vi "Decode and Update.vi"(8 "error in":errorcluster, 9 "WiBCI16T Data":T1 {"Reg Map"."ADS2" format="%x"; "Reg Map"."ADS1" format="%x"}, 10 "data in":string, 11 "Data Valid ?":bool) -> (0 "error out":errorcluster, 3 "WiBCI16T Data out":T1 {"Reg Map"."ADS2" format="%x"; "Reg Map"."ADS1" format="%x"})   [LabVIEW 2019, in "Acquisition.lvlib"]
uses:
  Acquisition.lvlib
  WiBCI16T_Data.ctl
  WiBCI16T_Status.ctl
  Reg_Map.ctl
panel:
  out "substring":string
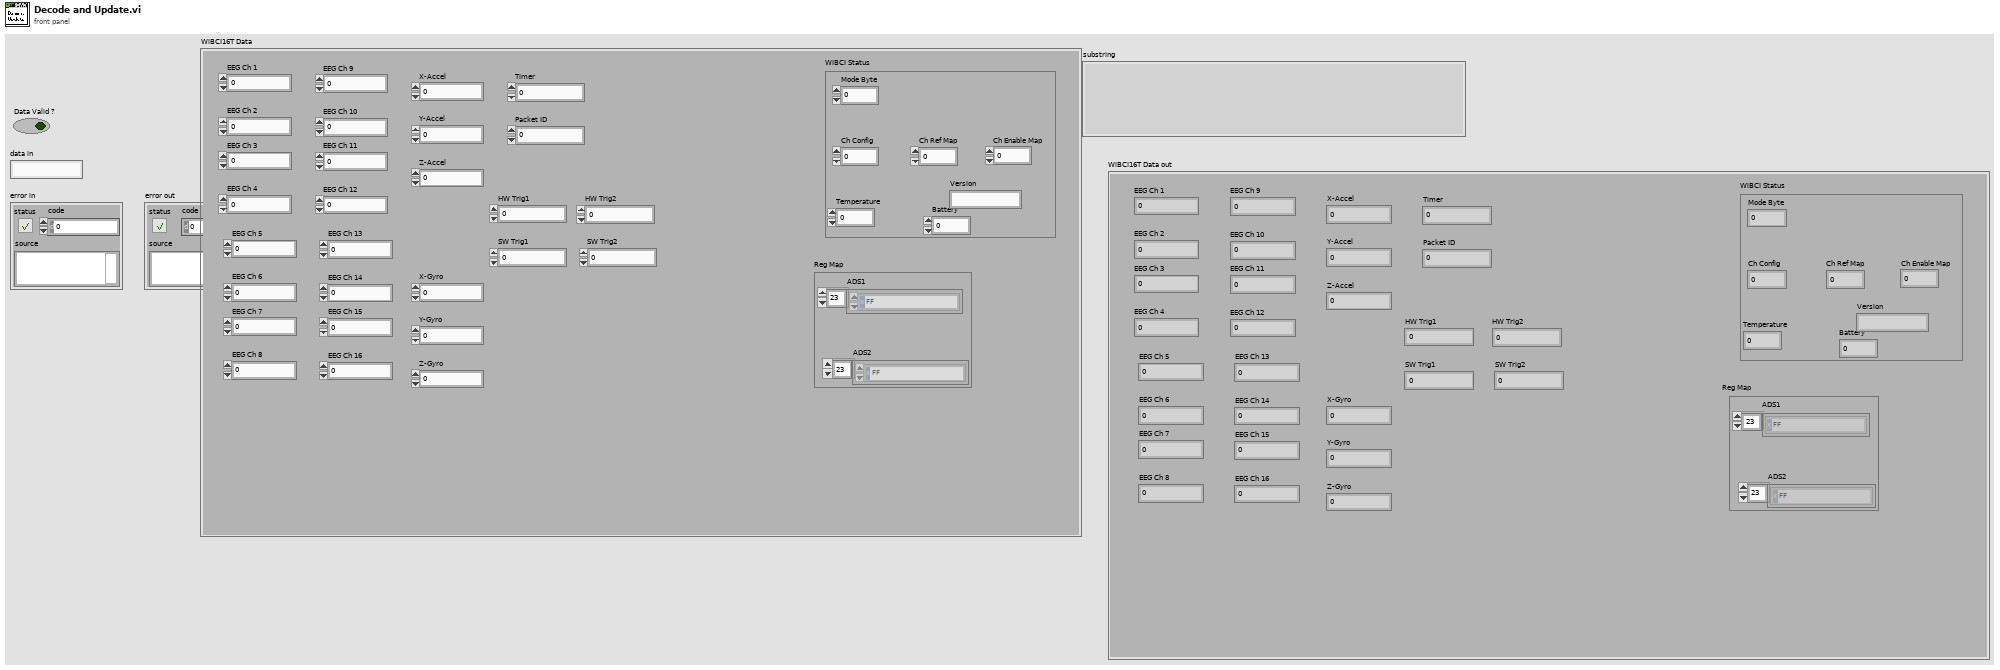
[diagram p1: front panel]
types:
  T1 = typedef "Acquisition.lvlib/WiBCI16T_Data.ctl" = cluster{"EEG Ch 1":dbl, "EEG Ch 2":dbl, "EEG Ch 3":dbl, "EEG Ch 4":dbl, "EEG Ch 5":dbl, "EEG Ch 6":dbl, "EEG Ch 7":dbl, "EEG Ch 8":dbl, "EEG Ch 9":dbl, "EEG Ch 10":dbl, "EEG Ch 11":dbl, "EEG Ch 12":dbl, "EEG Ch 13":dbl, "EEG Ch 14":dbl, "EEG Ch 15":dbl, "EEG Ch 16":dbl, "X-Accel":i16, "Y-Accel":i16, "Z-Accel":i16, "X-Gyro":i16, "Y-Gyro":i16, "Z-Gyro":i16, "Timer":u32, "Packet ID":u32, "HW Trig1":u8, "SW Trig1":i8, "HW Trig2":u8, "SW Trig2":i8, "WiBCI Status":T2, "Reg Map":T3}
  T2 = typedef "Acquisition.lvlib/WiBCI16T_Status.ctl" = cluster{"Mode Byte":u8, "Ch Config":u8, "Ch Ref Map":u16, "Ch Enable Map":u16, "Temperature":sgl, "Battery":u8, "Version":string}
  T3 = typedef "Acquisition.lvlib/Reg_Map.ctl" = cluster{"ADS1":u8[], "ADS2":u8[]}
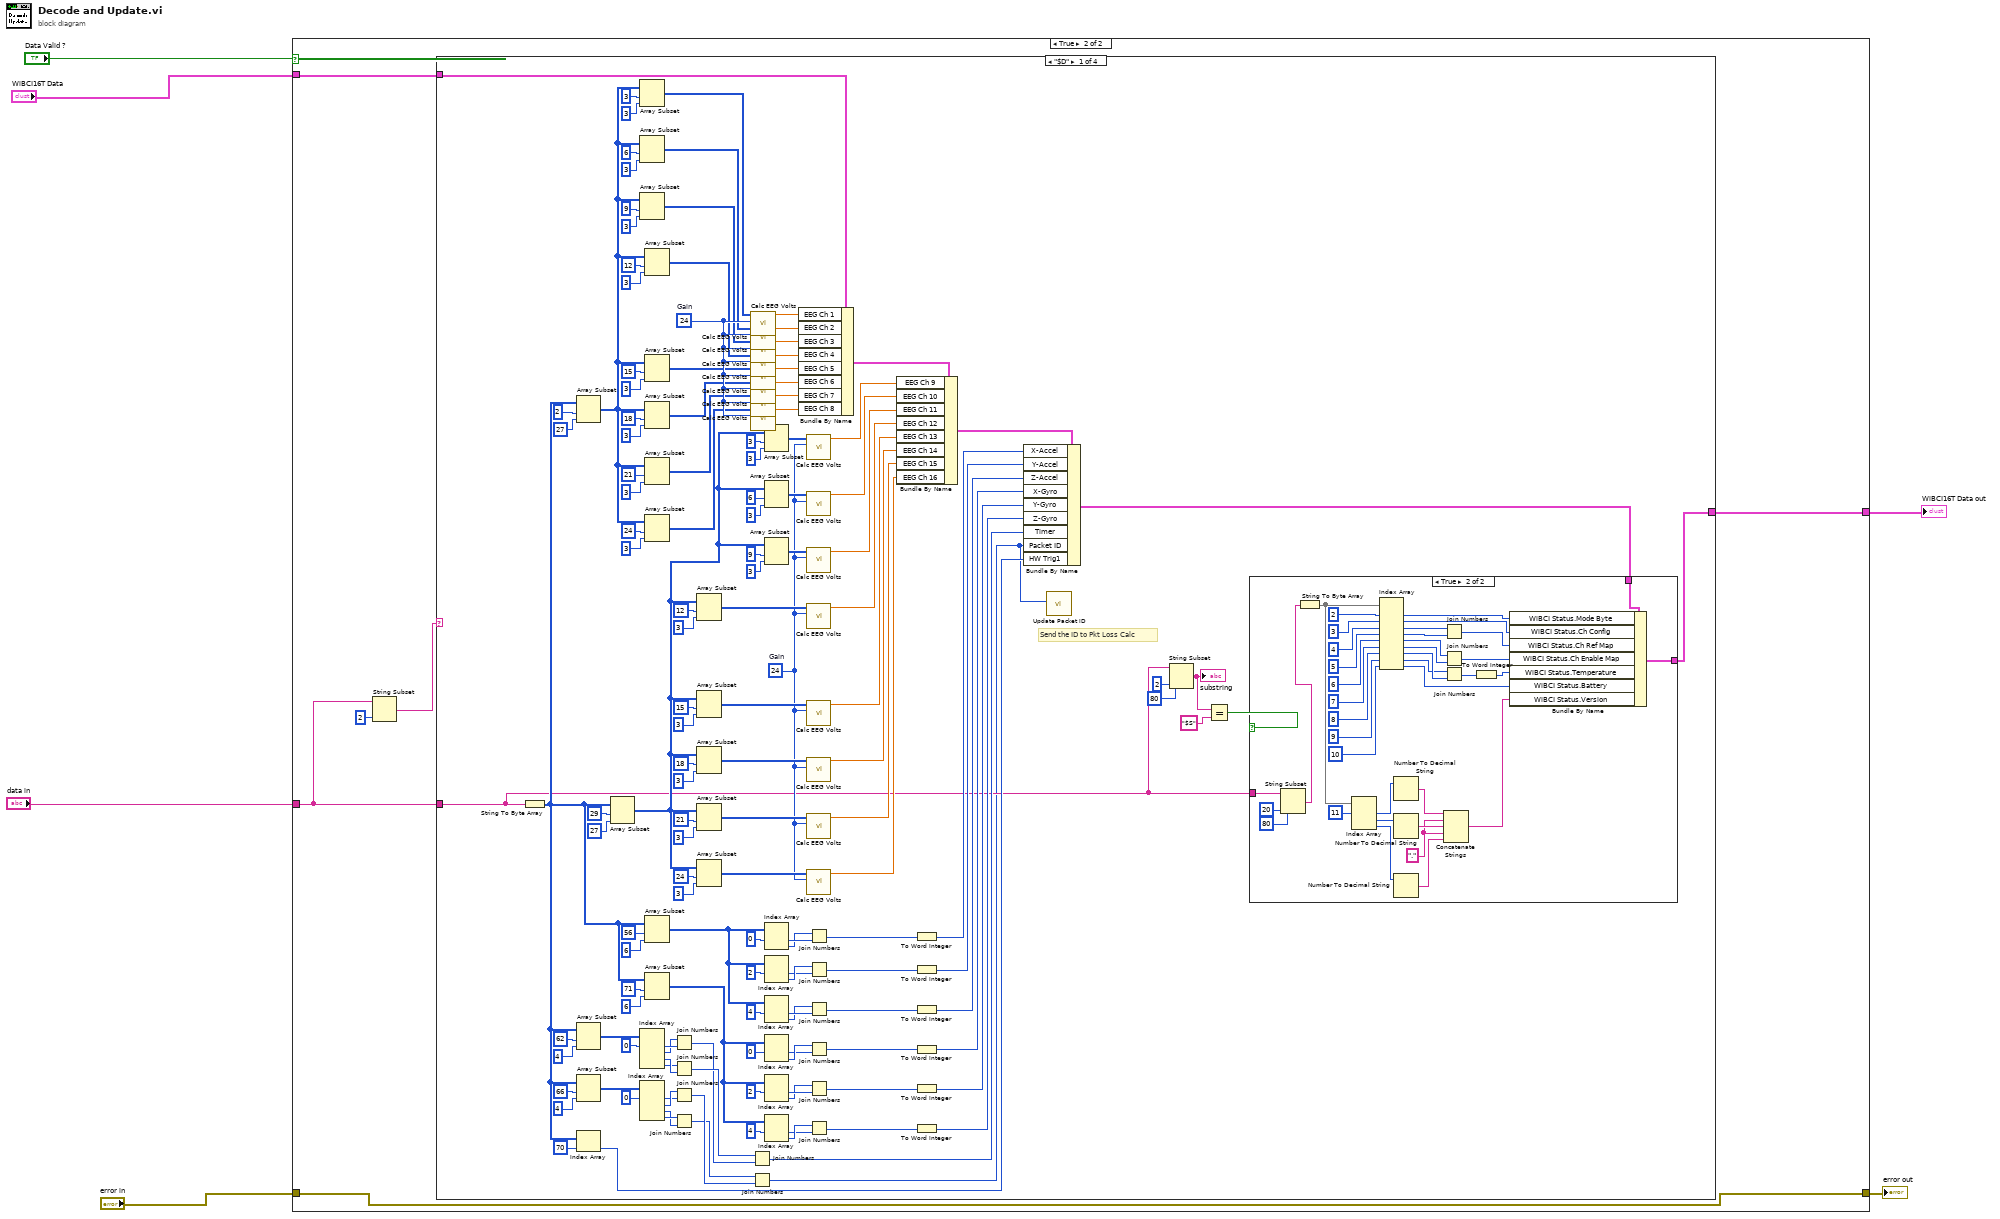
[diagram p0: block diagram]
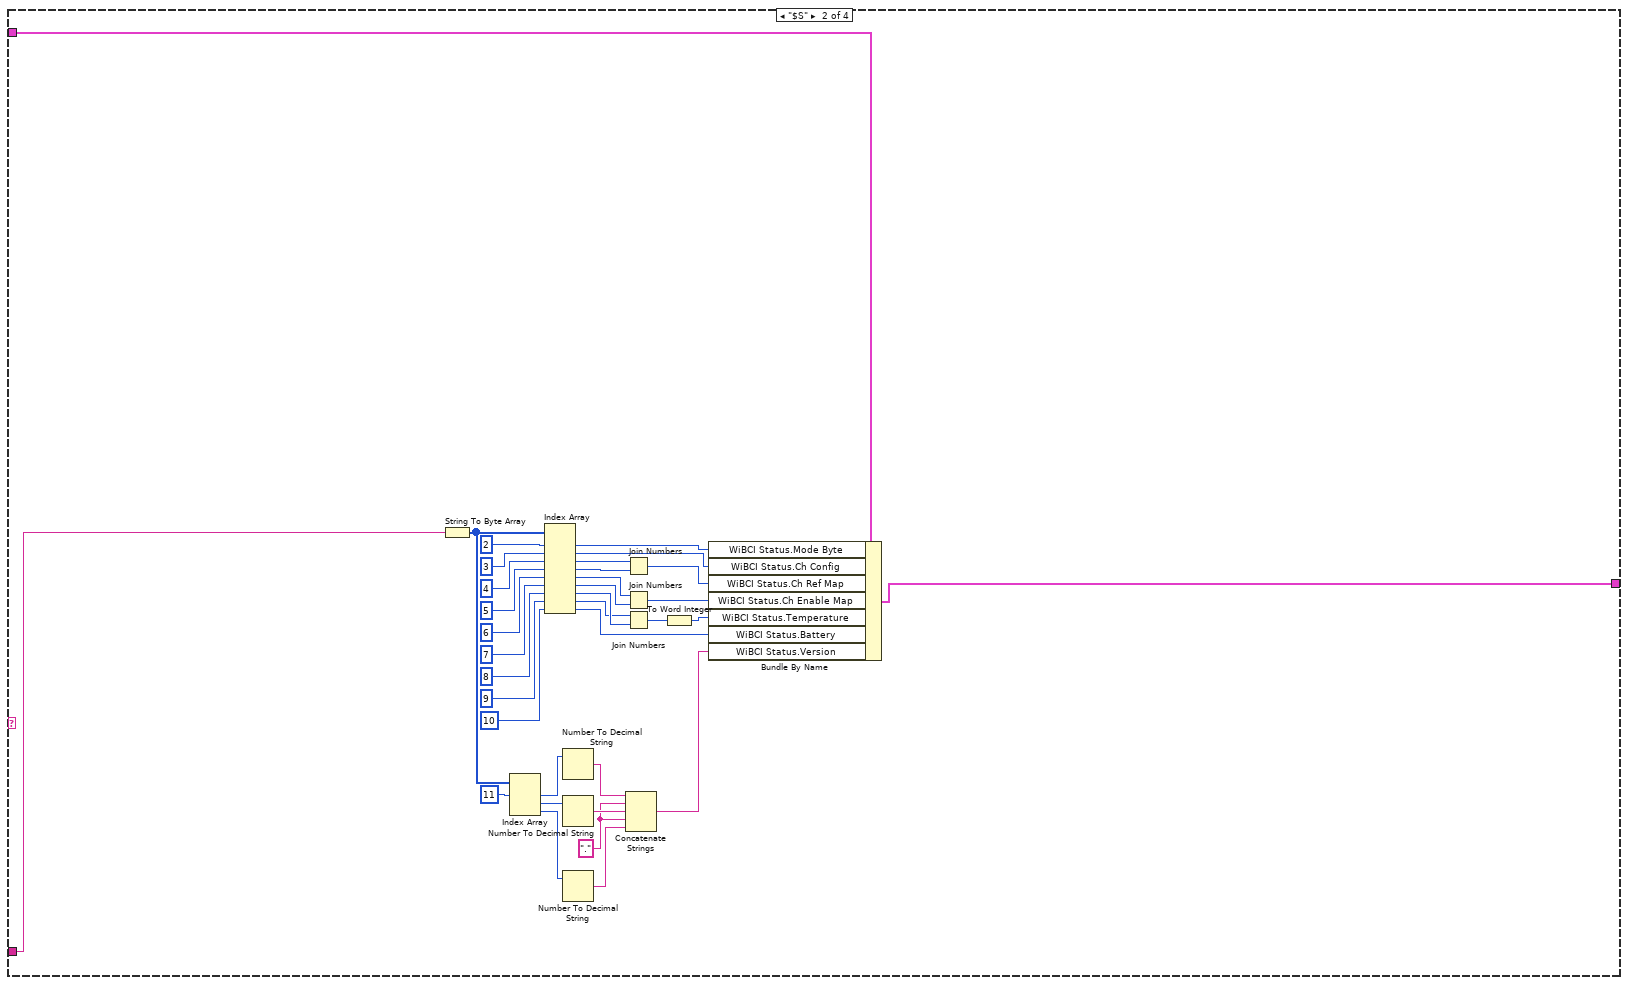
[diagram p4: hidden frame]
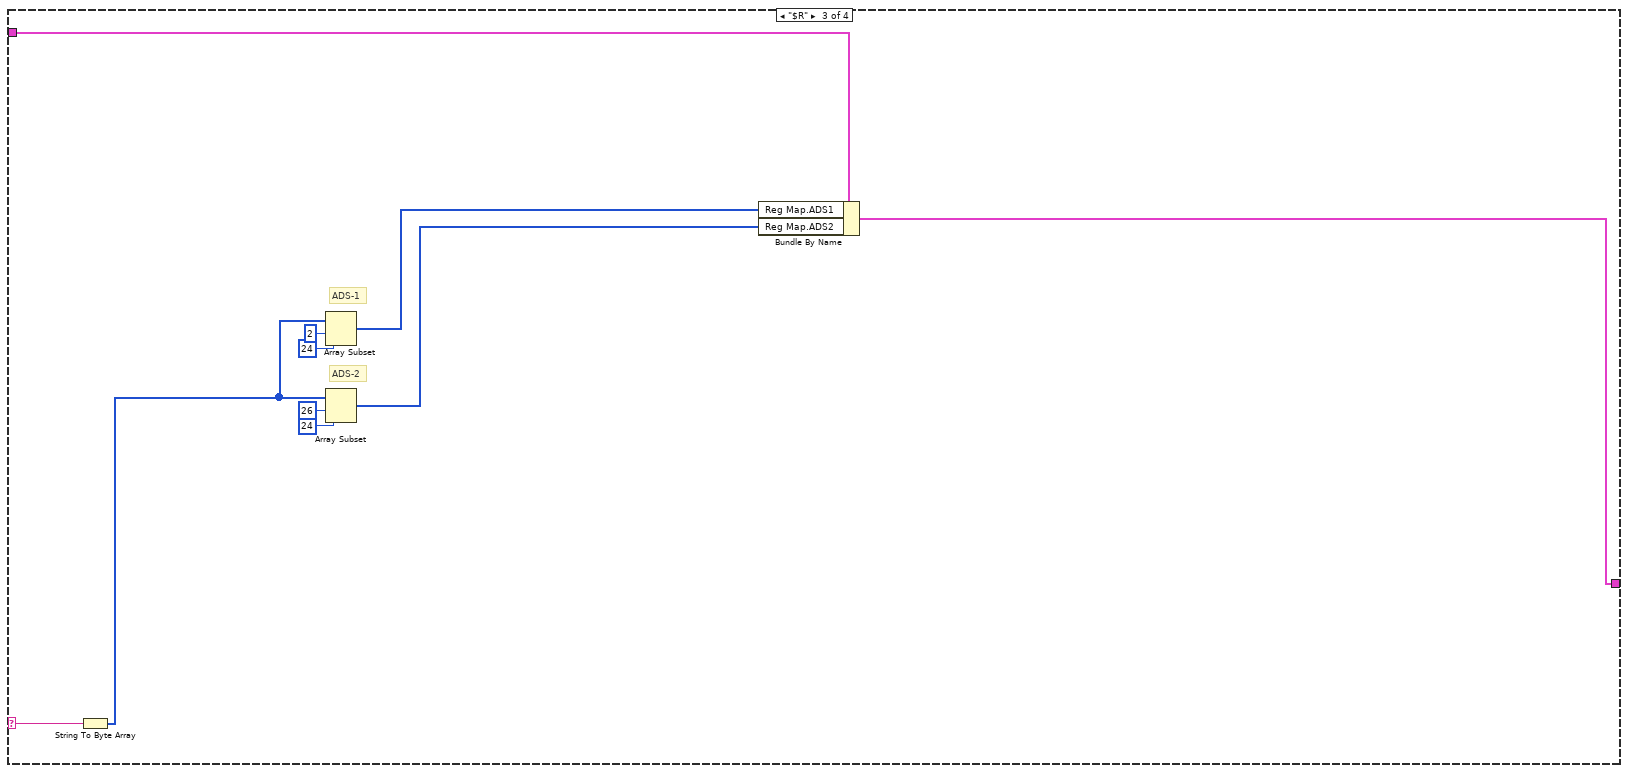
[diagram p5: hidden frame]
diagram:
  n1 = case shown="True" "Data Valid ?" {
    tunnel: "error in" -> [w8 w12]
    tunnel: [w8 w12] -> w5
    tunnel: "data in" -> [_ w10]
    tunnel: "WiBCI16T Data" -> [w7 w14]
    tunnel: [w7 w13] -> w1
    frame False {
    }
    frame True {
      n2 = String Subset(string=w10, length (rest)=2 ("length (rest)")) -> (substring=w9:string)  [unwired: 1 in]
      n3 = case shown="\"$D\"" w9 {
        selector: w9 -> [_ _ w236 _]
        tunnel: w14 -> [w128 w232 w242 w243]
        tunnel: [w16 w231 w241 w243] -> w13
        tunnel: w10 -> [w18 w198 _ _]
        frame "$D" {
          w103 = u8 24  # Gain
          w137 = u8 24  # Gain
          # "Send the ID to Pkt Loss Calc"
          n4 = String To Byte Array(string=w18) -> (unsigned byte array=w26:u8[])
          n5 = Array Subset(array=w26, index=2, length=27) -> (w138:u8[])
          n6 = Array Subset(array=w26, index=62, length=4) -> (w45:u8[])
          n7 = Array Subset(array=w26, index=66, length=4) -> (w30:u8[])
          n8 = Index Array(array=w26, index=70) -> (element=w24:u8)
          n9 = Array Subset(array=w26, index=29, length=27) -> (w85:u8[])
          n10 = Array Subset(array=w138, index=3, length=3) -> (w136:u8[])
          n11 = Array Subset(array=w138, index=6, length=3) -> (w135:u8[])
          n12 = Array Subset(array=w138, index=9, length=3) -> (w134:u8[])
          n13 = Index Array(array=w45, index #1=0 ("index")) -> (element #1=w43:u8, element #2=w42:u8, element #3=w41:u8, element #4=w40:u8)  [unwired: 3 in]
          n14 = Index Array(array=w30, index #1=0 ("index")) -> (element #1=w32:u8, element #2=w33:u8, element #3=w34:u8, element #4=w35:u8)  [unwired: 3 in]
          n15 = Array Subset(array=w138, index=12, length=3) -> (w133:u8[])
          n16 = Array Subset(array=w138, index=15, length=3) -> (w132:u8[])
          n17 = Array Subset(array=w138, index=18, length=3) -> (w131:u8[])
          n18 = Array Subset(array=w138, index=21, length=3) -> (w130:u8[])
          n19 = Array Subset(array=w138, index=24, length=3) -> (w129:u8[])
          n20 = Array Subset(array=w26, index=56, length=6) -> (w69:u8[])
          n21 = Array Subset(array=w26, index=71, length=6) -> (w65:u8[])
          n22 = Join Numbers(hi=w42, lo=w43) -> ((hi.lo)=w38:u16)
          n23 = Join Numbers(hi=w40, lo=w41) -> ((hi.lo)=w39:u16)
          n24 = Join Numbers(hi=w33, lo=w32) -> ((hi.lo)=w37:u16)
          n25 = Join Numbers(hi=w35, lo=w34) -> ((hi.lo)=w36:u16)
          n26 = Array Subset(array=w85, index=12, length=3) -> (w107:u8[])
          n27 = Array Subset(array=w85, index=15, length=3) -> (w108:u8[])
          n28 = Array Subset(array=w85, index=18, length=3) -> (w109:u8[])
          n29 = Array Subset(array=w85, index=21, length=3) -> (w110:u8[])
          n30 = Array Subset(array=w85, index=24, length=3) -> (w111:u8[])
          n31 = Join Numbers(hi=w39, lo=w38) -> ((hi.lo)=w27:u32)
          n32 = Join Numbers(hi=w36, lo=w37) -> ((hi.lo)=w15:u32)
          n33 = call "Calc EEG Volts.vi"("Gain"=w137, "Array"=w136) -> ("Volts"=w127:dbl)  [unwired: 9 in]
          n34 = call "Calc EEG Volts.vi"("Gain"=w137, "Array"=w135) -> ("Volts"=w126:dbl)  [unwired: 9 in]
          n35 = call "Calc EEG Volts.vi"("Gain"=w137, "Array"=w134) -> ("Volts"=w125:dbl)  [unwired: 9 in]
          n36 = call "Calc EEG Volts.vi"("Gain"=w137, "Array"=w133) -> ("Volts"=w124:dbl)  [unwired: 9 in]
          n37 = call "Calc EEG Volts.vi"("Gain"=w137, "Array"=w132) -> ("Volts"=w123:dbl)  [unwired: 9 in]
          n38 = call "Calc EEG Volts.vi"("Gain"=w137, "Array"=w131) -> ("Volts"=w122:dbl)  [unwired: 9 in]
          n39 = call "Calc EEG Volts.vi"("Gain"=w137, "Array"=w130) -> ("Volts"=w121:dbl)  [unwired: 9 in]
          n40 = call "Calc EEG Volts.vi"("Gain"=w137, "Array"=w129) -> ("Volts"=w120:dbl)  [unwired: 9 in]
          n41 = Array Subset(array=w85, index=3, length=3) -> (w104:u8[])
          n42 = Array Subset(array=w85, index=6, length=3) -> (w105:u8[])
          n43 = Array Subset(array=w85, index=9, length=3) -> (w106:u8[])
          n44 = Index Array(array=w69, index #1=0 ("index")) -> (element #1=w80:u8, element #2=w79:u8)  [unwired: 1 in]
          n45 = Index Array(array=w69, index #1=2 ("index")) -> (element #1=w75:u8, element #2=w76:u8)  [unwired: 1 in]
          n46 = Index Array(array=w69, index #1=4 ("index")) -> (element #1=w72:u8, element #2=w71:u8)  [unwired: 1 in]
          n47 = Index Array(array=w65, index #1=0 ("index")) -> (element #1=w54:u8, element #2=w55:u8)  [unwired: 1 in]
          n48 = Index Array(array=w65, index #1=2 ("index")) -> (element #1=w59:u8, element #2=w58:u8)  [unwired: 1 in]
          n49 = Index Array(array=w65, index #1=4 ("index")) -> (element #1=w62:u8, element #2=w63:u8)  [unwired: 1 in]
          n50 = Bundle By Name(cluster=w128, "EEG Ch 1"=w127, "EEG Ch 2"=w126, "EEG Ch 3"=w125, "EEG Ch 4"=w124, "EEG Ch 5"=w123, "EEG Ch 6"=w122, "EEG Ch 7"=w121, "EEG Ch 8"=w120) -> (w86:T1)
          n51 = call "Calc EEG Volts.vi"("Gain"=w103, "Array"=w104) -> ("Volts"=w112:dbl)  [unwired: 9 in]
          n52 = call "Calc EEG Volts.vi"("Gain"=w103, "Array"=w105) -> ("Volts"=w113:dbl)  [unwired: 9 in]
          n53 = call "Calc EEG Volts.vi"("Gain"=w103, "Array"=w106) -> ("Volts"=w114:dbl)  [unwired: 9 in]
          n54 = call "Calc EEG Volts.vi"("Gain"=w103, "Array"=w107) -> ("Volts"=w115:dbl)  [unwired: 9 in]
          n55 = call "Calc EEG Volts.vi"("Gain"=w103, "Array"=w108) -> ("Volts"=w116:dbl)  [unwired: 9 in]
          n56 = call "Calc EEG Volts.vi"("Gain"=w103, "Array"=w109) -> ("Volts"=w117:dbl)  [unwired: 9 in]
          n57 = call "Calc EEG Volts.vi"("Gain"=w103, "Array"=w110) -> ("Volts"=w118:dbl)  [unwired: 9 in]
          n58 = call "Calc EEG Volts.vi"("Gain"=w103, "Array"=w111) -> ("Volts"=w119:dbl)  [unwired: 9 in]
          n59 = Join Numbers(hi=w79, lo=w80) -> ((hi.lo)=w78:u16)
          n60 = Join Numbers(hi=w76, lo=w75) -> ((hi.lo)=w77:u16)
          n61 = Join Numbers(hi=w71, lo=w72) -> ((hi.lo)=w70:u16)
          n62 = Join Numbers(hi=w55, lo=w54) -> ((hi.lo)=w56:u16)
          n63 = Join Numbers(hi=w58, lo=w59) -> ((hi.lo)=w57:u16)
          n64 = Join Numbers(hi=w63, lo=w62) -> ((hi.lo)=w64:u16)
          n65 = Bundle By Name(cluster=w86, "EEG Ch 9"=w112, "EEG Ch 10"=w113, "EEG Ch 11"=w114, "EEG Ch 12"=w115, "EEG Ch 13"=w116, "EEG Ch 14"=w117, "EEG Ch 15"=w118, "EEG Ch 16"=w119) -> (w84:T1)
          n66 = To Word Integer(number=w78) -> (16bit integer=w68:i16)
          n67 = To Word Integer(number=w77) -> (16bit integer=w67:i16)
          n68 = To Word Integer(number=w70) -> (16bit integer=w66:i16)
          n69 = To Word Integer(number=w56) -> (16bit integer=w50:i16)
          n70 = To Word Integer(number=w57) -> (16bit integer=w49:i16)
          n71 = To Word Integer(number=w64) -> (16bit integer=w48:i16)
          n72 = Bundle By Name(cluster=w84, "X-Accel"=w68, "Y-Accel"=w67, "Z-Accel"=w66, "X-Gyro"=w50, "Y-Gyro"=w49, "Z-Gyro"=w48, "Timer"=w27, "Packet ID"=w15, "HW Trig1"=w24) -> (w17:T1)
          n73 = call "Update Packet ID.vi"("Packet ID"=w15) -> ()  [unwired: 10 in, 1 out]
          n74 = String Subset(string=w18, offset (0)=80, length (rest)=2 ("length (rest)")) -> (substring=w21:string)
          "substring" <- w21
          n75 = Equal?(x=w21, y="$S") -> (x = y?=w19:bool)
          n76 = case shown="True" w19 {
            tunnel: w18 -> [_ w161]
            tunnel: w17 -> [w159 w165]
            tunnel: [w159 w164] -> w16
            frame False {
            }
            frame True {
              w190 = "."
              n77 = String Subset(string=w161, offset (0)=80, length (rest)=20 ("length (rest)")) -> (substring=w160:string)
              n78 = String To Byte Array(string=w160) -> (unsigned byte array=w167:u8[])
              n79 = Index Array(array=w167, index #1=11 ("index")) -> (element #1=w196:u8, element #2=w195:u8, element #3=w194:u8)  [unwired: 2 in]
              n80 = Index Array(array=w167, index #1=2 ("index"), index #2=3 ("index"), index #3=4 ("index"), index #4=5 ("index"), index #5=6 ("index"), index #6=7 ("index"), index #7=8 ("index"), index #8=9 ("index"), index #9=10 ("index")) -> (element #1=w188:u8, element #2=w186:u8, element #3=w180:u8, element #4=w179:u8, element #5=w178:u8, element #6=w177:u8, element #7=w173:u8, element #8=w172:u8, element #9=w168:u8)
              n81 = Number To Decimal String(number=w196) -> (decimal integer string=w193:string)  [unwired: 1 in]
              n82 = Number To Decimal String(number=w195) -> (decimal integer string=w192:string)  [unwired: 1 in]
              n83 = Number To Decimal String(number=w194) -> (decimal integer string=w191:string)  [unwired: 1 in]
              n84 = Join Numbers(hi=w180, lo=w179) -> ((hi.lo)=w176:u16)
              n85 = Join Numbers(hi=w178, lo=w177) -> ((hi.lo)=w175:u16)
              n86 = Join Numbers(hi=w172, lo=w173) -> ((hi.lo)=w171:u16)
              n87 = Concatenate Strings(w193, w190, w192, w190, w191) -> (w166:string)
              n88 = To Word Integer(number=w171) -> (16bit integer=w170:i16)
              n89 = Bundle By Name(cluster=w165, "WiBCI Status.Mode Byte"=w188, "WiBCI Status.Ch Config"=w186, "WiBCI Status.Ch Ref Map"=w176, "WiBCI Status.Ch Enable Map"=w175, "WiBCI Status.Temperature"=w170, "WiBCI Status.Battery"=w168, "WiBCI Status.Version"=w166) -> (w164:T1)
            }
          }
        }
        frame "$S" {
          w223 = "."
          n90 = String To Byte Array(string=w198) -> (unsigned byte array=w200:u8[])
          n91 = Index Array(array=w200, index #1=11 ("index")) -> (element #1=w229:u8, element #2=w228:u8, element #3=w227:u8)  [unwired: 2 in]
          n92 = Index Array(array=w200, index #1=2 ("index"), index #2=3 ("index"), index #3=4 ("index"), index #4=5 ("index"), index #5=6 ("index"), index #6=7 ("index"), index #7=8 ("index"), index #8=9 ("index"), index #9=10 ("index")) -> (element #1=w221:u8, element #2=w219:u8, element #3=w213:u8, element #4=w212:u8, element #5=w211:u8, element #6=w210:u8, element #7=w206:u8, element #8=w205:u8, element #9=w201:u8)
          n93 = Number To Decimal String(number=w229) -> (decimal integer string=w226:string)  [unwired: 1 in]
          n94 = Number To Decimal String(number=w228) -> (decimal integer string=w225:string)  [unwired: 1 in]
          n95 = Number To Decimal String(number=w227) -> (decimal integer string=w224:string)  [unwired: 1 in]
          n96 = Join Numbers(hi=w213, lo=w212) -> ((hi.lo)=w209:u16)
          n97 = Join Numbers(hi=w211, lo=w210) -> ((hi.lo)=w208:u16)
          n98 = Join Numbers(hi=w205, lo=w206) -> ((hi.lo)=w204:u16)
          n99 = Concatenate Strings(w226, w223, w225, w223, w224) -> (w199:string)
          n100 = To Word Integer(number=w204) -> (16bit integer=w203:i16)
          n101 = Bundle By Name(cluster=w232, "WiBCI Status.Mode Byte"=w221, "WiBCI Status.Ch Config"=w219, "WiBCI Status.Ch Ref Map"=w209, "WiBCI Status.Ch Enable Map"=w208, "WiBCI Status.Temperature"=w203, "WiBCI Status.Battery"=w201, "WiBCI Status.Version"=w199) -> (w231:T1)
        }
        frame "$R" {
          # "ADS-2"
          # "ADS-1"
          n102 = String To Byte Array(string=w236) -> (unsigned byte array=w235:u8[])
          n103 = Array Subset(array=w235, index=2, length=24) -> (w234:u8[])
          n104 = Array Subset(array=w235, index=26, length=24) -> (w233:u8[])
          n105 = Bundle By Name(cluster=w242, "Reg Map.ADS1"=w234, "Reg Map.ADS2"=w233) -> (w241:T1)
        }
        frame "GARBAGE", Default {
        }
      }
    }
  }
  "error out" <- w5
  "WiBCI16T Data out" <- w1
